vi "Threshold with Hysteresis 2.vi"(6 "Hystersis":dbl=10.0, 7 "Threshold":dbl=60.0, 8 "Input Dif":dbl(slide)=70.0 step=1.0 scale=-1000.0..1000.0 scale format="%1.1f") -> (0 "Below Theshold Hyst":bool, 1 "Threshold":bool, 2 "Power":bool, 3 "Out Dif Last":dbl)   [LabVIEW 2012]
doc: "Use this template to build a standard state machine design pattern. Each state executes code and determines which state to transition to. Contrast this design pattern with the User Interface Event Handler pattern, in which code executes in response to user actions. Contrast this design pattern also with the Queued Message Handler pattern, in which each message handling code can queue zero or more new messages."
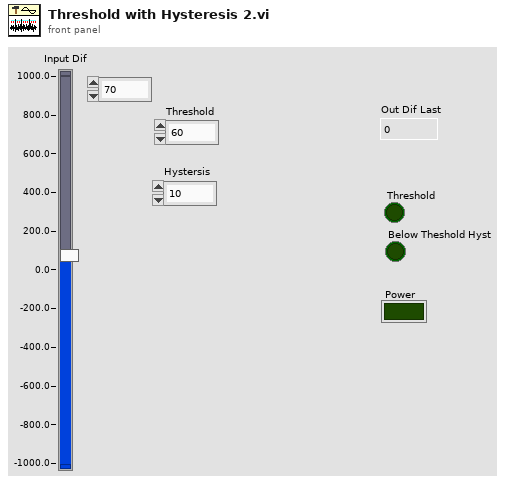
[diagram p1: front panel]
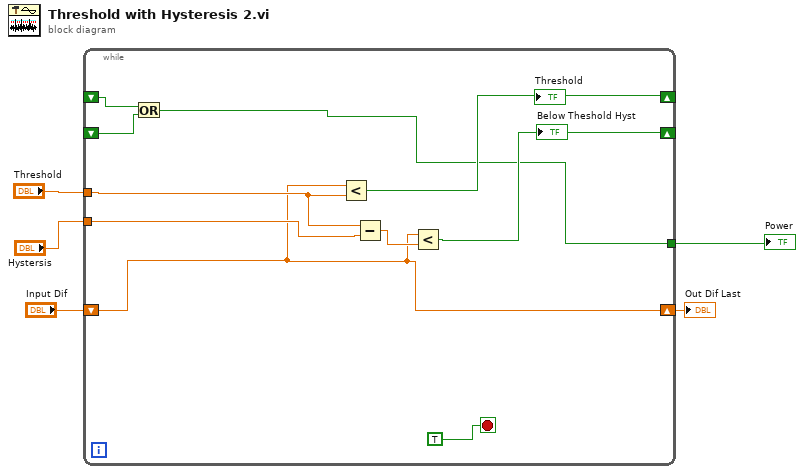
[diagram p0: block diagram]
diagram:
  n1 = while {
    tunnel: "Threshold" -> [w14]
    tunnel: "Hystersis" -> [w13]
    shift-right: [w10] -> _
    shift-left: _ -> [w9]
    shift-right: [w11] -> _
    shift-left: _ -> [w8]
    tunnel: [w7] -> w1
    shift-right: [w6] -> w2
    shift-left: "Input Dif" -> [w6]
    stop <- TRUE ("Boolean") stop-if-true
    n2 = Or(x=w9, y=w8) -> (x .or. y?=w7:bool)
    n3 = Less?(x=w6, y=w14) -> (x < y?=w10:bool)
    "Threshold" <- w10
    n4 = Subtract(x=w14, y=w13) -> (x-y=w12:dbl)
    n5 = Less?(x=w6, y=w12) -> (x < y?=w11:bool)
    "Below Theshold Hyst" <- w11
  }
  "Out Dif Last" <- w2
  "Power" <- w1
